vi "RP Read Subset TCP.vi"(6 "Bytes per sample":i32, 7 "Samples per trigger increment":i32=2, 8 "Error In":errorcluster, 9 "Post-trigger samples":u64=11534336 format="0x%x (%d)", 10 "Pre-trigger samples":i32=-100000 format="0x%x (%d)", 11 "connection ID":refnum<k5>) -> (0 "Error Out":errorcluster, 1 "Record start pos":u32=1, 2 "Data stream":string, 3 "connection ID out":refnum<k5>)   [LabVIEW 2016]
uses:
  RP Command.ctl
  RP Status Offsets.ctl
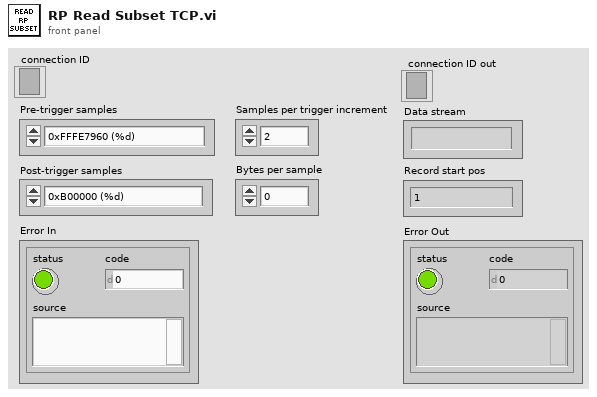
[diagram p1: front panel]
types:
  T1 = typedef "RP Status Offsets.ctl" = u16
  T2 = typedef "RP Command.ctl" = enum16{"Reset", "Read IDN", "Stop server", "Get status", "Get temperature", "Connect client", "Arm", "Software trigger", "Get whole buffer", "Get chunk", "System call", "Get config", "Set config", "Recieve data", "Recieve Calibartion", "Transmit data"}
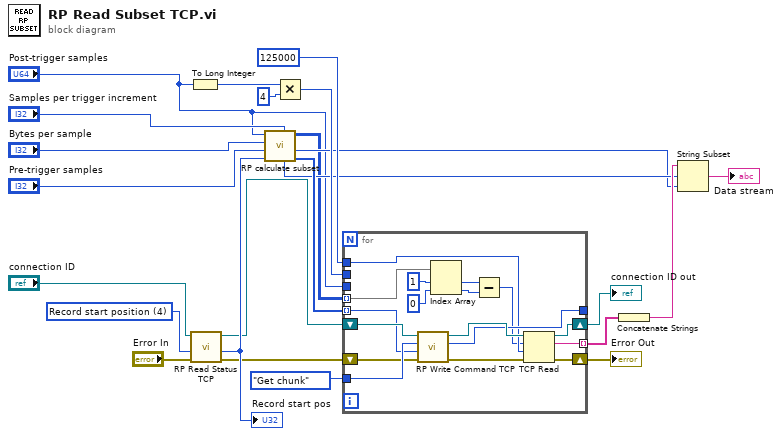
[diagram p0: block diagram]
diagram:
  w19 = T1 4 items=["Writer address"=0, "Record start position"=4, "Trig state etc."=8, "RxFIFO counter"=24, "TxFIFO counter"=28] ("Status offset")
  n1 = To Long Integer(number="Post-trigger samples") -> (32bit integer=w21:i32)
  n2 = call "RP Read Status TCP.vi"("Error In"="Error In", "Status offset"=w19, "connection ID"="connection ID") -> ("Error Out"=w9:errorcluster, "Status response"=w18:u32, "connection ID out"=w17:refnum<k5>)  [unwired: 6 in]
  "Record start pos" <- w18
  n3 = call "RP calculate subset.vi"("Samples per trigger increment"="Samples per trigger increment", "Trigger start position"=w18, "Pre-trigger samples"="Pre-trigger samples", "Bytes per sample"="Bytes per sample", "Post-trigger samples"="Post-trigger samples") -> ("Merged subsets"=w16:u64[], "record length"=w12:i32, "Subsets"=w5:i32[][], "pre-trigger trim"=w13:i32)  [unwired: 3 in]
  n4 = Multiply(x=w21, y=4) -> (x*y=w23:i32)
  n5 = for {
    tunnel: w23 -> [_]
    tunnel: RP_Command."Get chunk" ("Command number") -> [w41]
    tunnel: [w38] -> _
    tunnel: 125000 ("timeout ms (25000)") -> [w36]
    tunnel: "Post-trigger samples" -> [_]
    shift-right: [w35] -> w7
    shift-left: w9 -> [w34]
    shift-right: [w37] -> w10
    shift-left: w17 -> [w33]
    tunnel: w16 -> [w32] mode=indexing
    tunnel: [w31] -> w15 mode=indexing
    tunnel: w5 -> [w29] mode=indexing
    n6 = call "RP Write Command TCP.vi"("Error In"=w34, "Command payload"=w32, "Command number"=w41, "connection ID"=w33) -> ("Error Out"=w39:errorcluster, "bytes written"=w38:i32, "connection ID out"=w40:refnum<k5>)  [unwired: 5 in]
    n7 = Index Array(array=w29, index #1=1 ("index"), index #2=0 ("index")) -> (element #1=w28:i32, element #2=w27:i32)
    n8 = Subtract(x=w28, y=w27) -> (x-y=w26:i32)
    n9 = TCP Read(connection ID=w40, bytes to read=w26, error in (no error)=w39, 9:w36) -> (connection ID out=w37:refnum<k5>, data out=w31:string, error out=w35:errorcluster)  [unwired: 1 in]
  }
  "connection ID out" <- w10
  "Error Out" <- w7
  n10 = Concatenate Strings(w15) -> (w14:string)
  n11 = String Subset(string=w14, offset (0)=w13, length (rest)=w12) -> (substring=→"Data stream":string)
